vi "Interpolate Autobalance Data.vi"(8 "error in (no error)":errorcluster, 9 "Command Voltages":dbl[](array[numeric]), 10 "name or relative path":path, 11 "Actions":T1) -> (0 "error out":errorcluster, 2 "Servo Errors":dbl[](array[numeric]))   [LabVIEW 2009]
uses:
  Interpolate Actions.ctl
panel:
  out "size(s)":i32[](array[numeric])
  out "Autobalance Data":dbl[][](array[numeric])
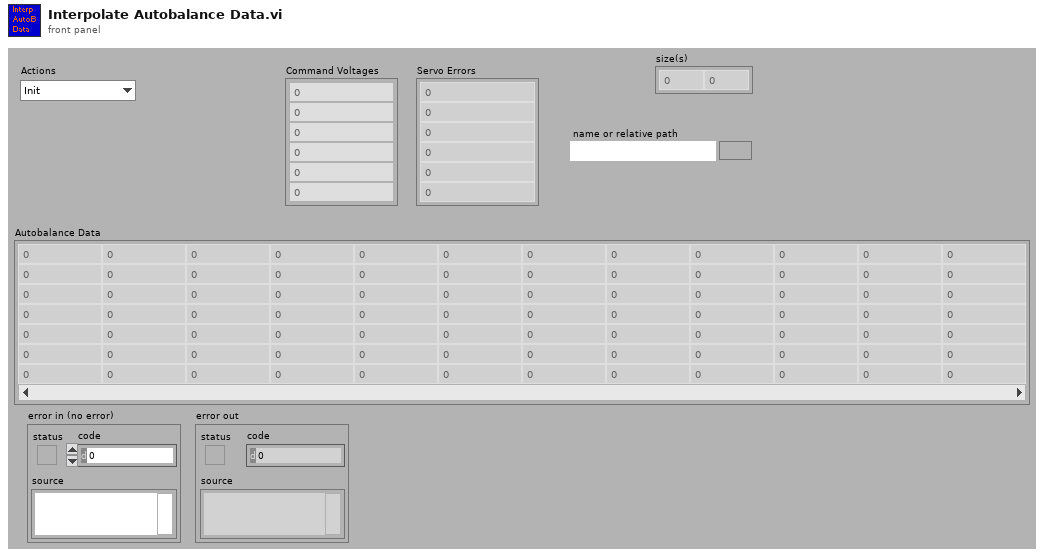
[diagram p1: front panel]
types:
  T1 = typedef "Interpolate Actions.ctl" = enum16{"Init", "Interpolate"}
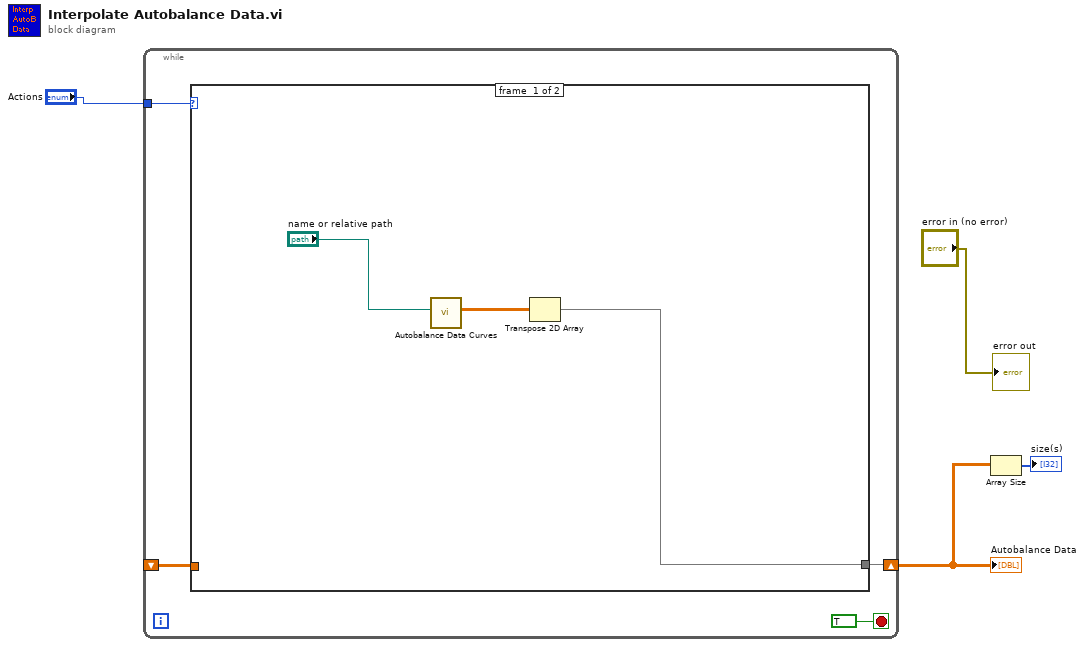
[diagram p0: block diagram]
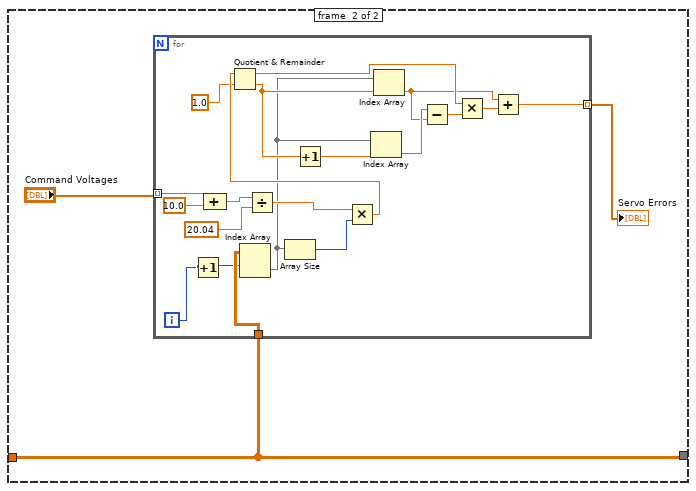
[diagram p2: hidden frame]
diagram:
  n1 = while {
    tunnel: "Actions" -> [w7]
    shift-right: [w6] -> w3
    shift-left: _ -> [w5]
    stop <- TRUE stop-if-true
    n2 = case shown="\"Init\"" w7 {
      tunnel: [w10 w14] -> w6
      tunnel: w5 -> [_ w14]
      frame #0 {
        n3 = call "Autobalance Data Curves.vi"("name or relative path"="name or relative path") -> ("all rows"=w11:dbl[][])  [unwired: 10 out]
        n4 = Transpose 2D Array(2D array=w11) -> (transposed array=w10:dbl[][])
      }
      frame #1 {
        n5 = for {
          tunnel: w14 -> [w34]
          tunnel: "Command Voltages" -> [w31] mode=indexing
          tunnel: [w20] -> w12 mode=indexing
          i -> [w32]
          n6 = Increment(x=w32) -> (x+1=w33:i32)
          n7 = Compound Arithmetic op=ADD(w31, 10.0 ("y")) -> (w29:dbl)
          n8 = Index Array(array=w34, index (row)=w33) -> (element=w22:dbl[])  [unwired: 1 in]
          n9 = Divide(x=w29, y=20.04) -> (x/y=w27:dbl)
          n10 = Array Size(array=w22) -> (size(s)=w26:i32)
          n11 = Multiply(x=w27, y=w26) -> (x*y=w25:dbl)
          n12 = Quotient & Remainder(x=w25, y=1.0) -> (x-y*floor(x/y)=w21:dbl, floor(x/y)=w23:dbl)
          n13 = Increment(x=w23) -> (x+1=w19:dbl)
          n14 = Index Array(array=w22, index=w19) -> (element=w18:dbl)
          n15 = Index Array(array=w22, index=w23) -> (element=w15:dbl)
          n16 = Subtract(x=w18, y=w15) -> (x-y=w17:dbl)
          n17 = Multiply(x=w21, y=w17) -> (x*y=w16:dbl)
          n18 = Add(x=w15, y=w16) -> (x+y=w20:dbl)
        }
        "Servo Errors" <- w12
      }
    }
  }
  "Autobalance Data" <- w3
  n19 = Array Size(array=w3) -> (size(s)=→"size(s)":i32[])
  "error out" <- "error in (no error)"
